vi "VI Package List to SBOM Components.vi"(8 "error in (no error)":errorcluster, 11 "VIP List in":T1[](array[typedef])) -> (0 "error out":errorcluster, 3 "SBOM Components out":refnum<class "CycloneDX Component.lvclass">[](array[class]))   [LabVIEW 2017, in "VIP SBOM Support.lvlib"]
doc: "Converts an array of VI Package information into an array of CycloneDX SBOM components."
uses:
  VIP SBOM Support.lvlib
  CycloneDX/CycloneDX Component/CycloneDX Component.lvclass
  <vilib>/JKI/VIPM API/command-line/support/Library Contents Cluster_vipm_api.ctl
  <vilib>/JKI/VIPM API/VIPM API_vipm_api.lvlib
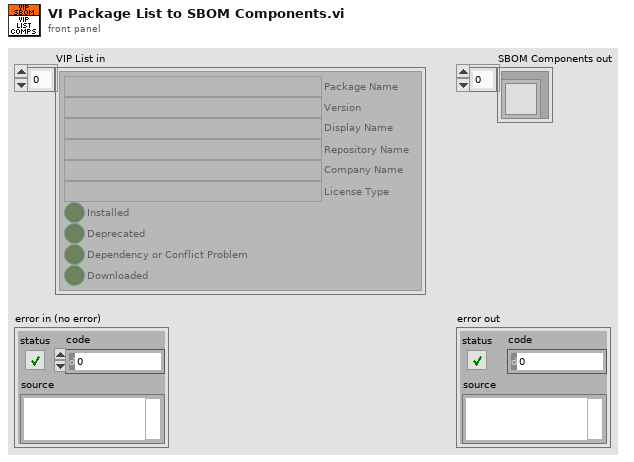
[diagram p1: front panel]
types:
  T1 = typedef "VIPM API_vipm_api.lvlib/Library Contents Cluster_vipm_api.ctl" = cluster{"Package Name":string, "Version":string, "Display Name":string, "Repository Name":string, "Company Name":string, "License Type":string, "Installed":bool, "Deprecated":bool, "Dependency or Conflict Problem":bool, "Downloaded":bool}
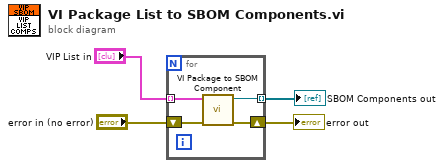
[diagram p0: block diagram]
diagram:
  n1 = for {
    tunnel: "VIP List in" -> [w8] mode=indexing
    shift-right: [w6] -> w3
    shift-left: "error in (no error)" -> [w7]
    tunnel: [w5] -> w4 mode=indexing
    n2 = call "VI Package to SBOM Component.vi"("error in (no error)"=w7, "VIP Information"=w8) -> ("error out"=w6:errorcluster, "CycloneDX Component"=w5:refnum<class "CycloneDX Component.lvclass">)  [unwired: 8 in]
  }
  "SBOM Components out" <- w4
  "error out" <- w3
